vi "Method_Const.vi"(4 "Value":dbl, 5 "Input A":refnum<class "Abs_Time.lvclass">) -> (1 "Result":refnum<class "Abs_Time.lvclass">)   [LabVIEW 2021, in "Add_Time.lvclass"]
uses:
  Add_Time.lvclass
  Abs_Types/Time/Abs_Time.lvclass
  C:/TSA/LV_Abstract/Source/Functions/Support/Function/Two Terminal/Time/AbsFunc_Two Term_Time.lvclass
  C:/Program Files (x86)/National Instruments/LabVIEW 2021/vi.lib/TSA/Abstract Data Classes/Abs_Types/Time/Abs_Time.lvclass
  Support/Function/Two Terminal/Time/AbsFunc_Two Term_Time.lvclass/AbsFunc_Two Term_Time.ctl
  Support/Function/Two Terminal/Time/Properties/Write Numeric A.vi
  Support/Function/Two Terminal/Time/Properties/Write Numeric B.vi
  Constants/Support/DBL/Const_DBL.lvclass
  C:/Program Files (x86)/National Instruments/LabVIEW 2021/vi.lib/TSA/Abstract Data Classes/Abs_Types/Numeric/Abs_Numeric.lvclass
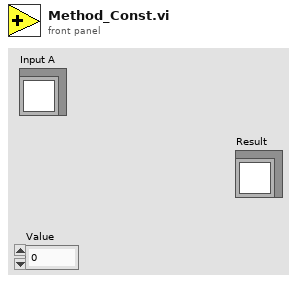
[diagram p1: front panel]
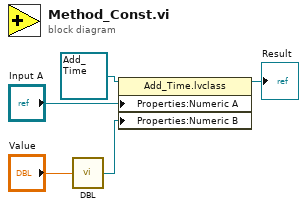
[diagram p0: block diagram]
diagram:
  n1 = call "DBL.vi"("Value"="Value") -> ("Constant"=w2:refnum<class "Const_DBL.lvclass">)  [unwired: 4 in]
  n2 = property class="Add_Time.lvclass"(reference=refnum<class "Add_Time.lvclass"> refnum ("Functions.lvlib:Numeric.lvlib:Add_DBL.lvclass"), "Properties:Numeric A"="Input A", "Properties:Numeric B"=w2) -> (reference out=→"Result":refnum<class "Add_Time.lvclass">)  [unwired: 1 in, 1 out]
